vi "json_Get_AddTopic.vi"(8 "error in":errorcluster, 11 "ReadCMD_0":string="{\"ID\": \"b9b762fb-e465-4f6a-bde5-995dda67237b\", \"TO\": \"845CF3525B43\", \"FROM\": \"C87F542F1180\", \"CMD\": 0, \"CONTENT\": [{\"HOSTNAME\": \"SI-AGT01\", \"MAC\": \"845CF3525B43\", \"IP\": \"172.20.10.10\", \"CENTER_NAME\": \"C87F542F1180\", \"ADD_TOPIC\": \"topic/PC/845CF3525B43\", \"REQ_ID\": \"38A46EA6-1EA1-4C1D-82A7-A29BD9BCAD25\"}], \"STATUS\": true, \"ERRCODE\": \"\", \"ERRMSG\": \"\", \"TIMESTAMP\": 1759035794") -> (0 "error out":errorcluster, 2 "AddTopic":string, 3 "Mac_Server":string)   [LabVIEW 2020]
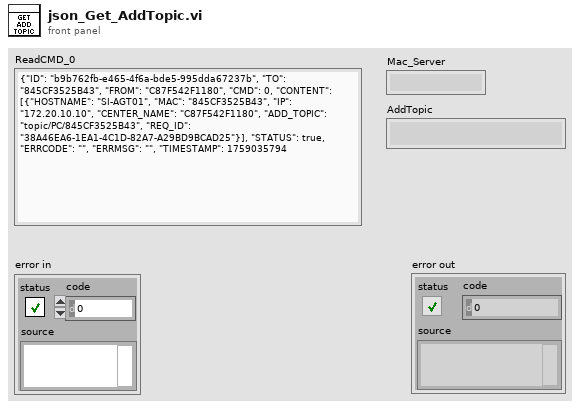
[diagram p1: front panel]
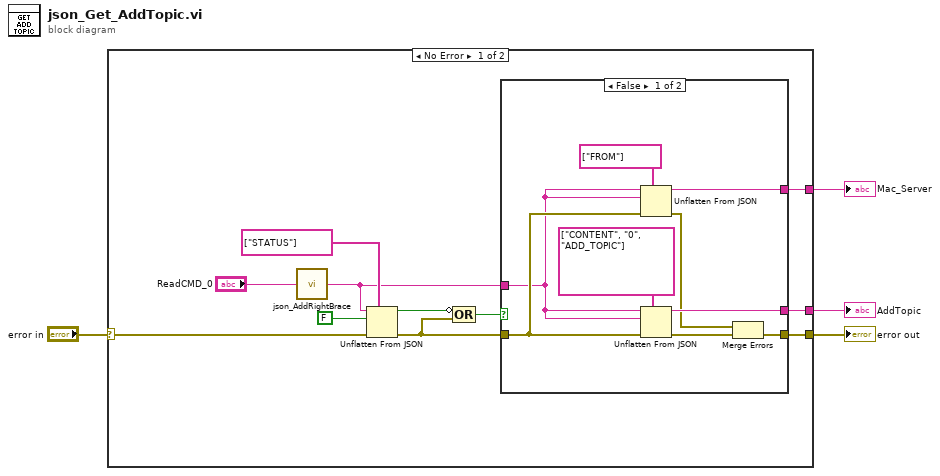
[diagram p0: block diagram]
diagram:
  n1 = case shown="No Error" "error in" {
    selector: "error in" -> [w6 w25]
    tunnel: [w9 w25] -> w4
    tunnel: [w8 _] -> w3
    tunnel: [w5 _] -> w1
    frame No Error {
      n2 = call "json_AddRightBrace.vi"("ReadCMD_0"="ReadCMD_0") -> ("+}"=w7:string)
      n3 = Unflatten From JSON(path=string[] ["STATUS"], JSON string=w7, type and defaults=FALSE, error in (no error)=w6) -> (value=w13:bool, error out=w12:errorcluster)  [unwired: 3 in]
      n4 = Compound Arithmetic op=OR(invert w13, w12) -> (w10:bool)
      n5 = case shown="False" w10 {
        tunnel: w12 -> [w19 _]
        tunnel: w7 -> [w18 _]
        tunnel: [w21 _] -> w9
        tunnel: [w23 _] -> w8
        tunnel: [w16 _] -> w5
        frame False {
          n6 = Unflatten From JSON(path=string[] ["FROM"], JSON string=w18, type and defaults=w18, error in (no error)=w19) -> (value=w16:string, error out=w20:errorcluster)  [unwired: 3 in]
          n7 = Unflatten From JSON(path=string[] ["CONTENT", "0", "ADD_TOPIC"], JSON string=w18, type and defaults=w18, error in (no error)=w19) -> (value=w23:string, error out=w22:errorcluster)  [unwired: 3 in]
          n8 = Merge Errors(w20, w22) -> (w21:errorcluster)
        }
        frame True {
        }
      }
    }
    frame Error {
    }
  }
  "error out" <- w4
  "AddTopic" <- w3
  "Mac_Server" <- w1
